vi "PC Main.vi"() -> ()   [LabVIEW 2016]
panel:
  in  "pause":bool
  in  "Stop Button":bool
  in  "stop \"RT Main\"":bool
  out "LEDb":bool
  out "LEDa":bool
  out "paused":bool
  in  "loop time [ms]":u32(slide)=100 scale=10.0..1000.0
  # "PC HMI"
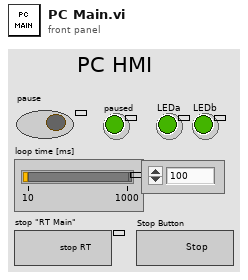
[diagram p1: front panel]
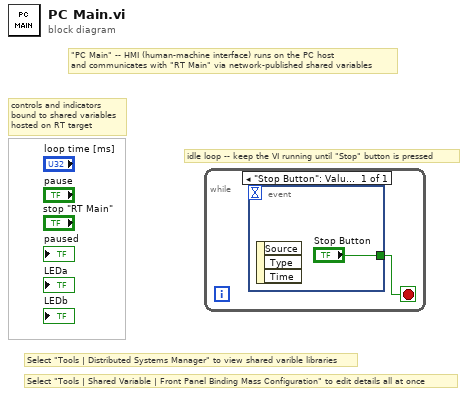
[diagram p0: block diagram]
diagram:
  # "Select \"Tools | Shared Variable | Front Panel Binding Mass Configuration\" to edit details all at once"
  # "Select \"Tools | Distributed Systems Manager\" to view shared varible libraries"
  # "controls and indicators\nbound to shared variables\nhosted on RT target"
  # "idle loop -- keep the VI running until \"Stop\" button is pressed"
  # "\"PC Main\" -- HMI (human-machine interface) runs on the PC host\nand communicates with \"RT Main\" via network-published shared variables"
  n1 = while {
    stop <- w1 stop-if-true
    n2 = event shown="[0] \"Stop Button\": Value Change" {
      selector: _ -> [_]
      dyn-events: _ -> [_]
      timeout: _ -> [_]
      tunnel: ["Stop Button"] -> w1
      event "Stop Button": Value Change {
        n3 = event-data() -> ()  [unwired: 1 in, 3 out]
      }
    }
  }
